vi "Create Channel Configuration.vi"(4 "non-random type (DBL)":T1=enum."DBL", 6 "random types? (F)":bool, 7 "base channel name (channel)":string="channel", 11 "channel count":i32) -> (2 "buffer size":u64, 3 "channel configurations":T2[](array[typedef]) {"buffer offset" format="%d bytes"})   [LabVIEW 2017]
uses:
  Builds/Data Sharing Framework/Current/Data Sharing Framework Core/DSF Core.lvlibp/DSF Configuration API/Public/Controls/DSF Engine Channel Configuration.ctl
  Builds/Data Sharing Framework/Current/Data Sharing Framework Core/DSF Core.lvlibp/DSF Configuration API/Public/Controls/DSF Data Type.ctl
  Builds/Data Sharing Framework/Current/Data Sharing Framework Core/DSF Core.lvlibp/DSF Configuration API/Public/Controls/DSF Settings Info.ctl
  Builds/Data Sharing Framework/Current/Data Sharing Framework Core/DSF Core.lvlibp
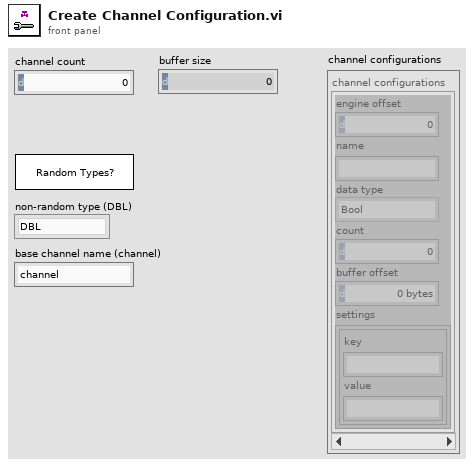
[diagram p1: front panel]
types:
  T1 = typedef "DSF Core.lvlibp/DSF Data Type.ctl" = enum8{"Bool", "SGL", "DBL", "I8", "I16", "I32", "I64", "U8", "U16", "U32", "U64"}
  T2 = typedef "DSF Core.lvlibp/DSF Engine Channel Configuration.ctl" = cluster{"engine offset":u64, "name":string, "data type":T1, "count":u64, "buffer offset":u64, "settings":T3}
  T3 = typedef "DSF Core.lvlibp/DSF Settings Info.ctl" = cluster{"key":string, "value":string}[]
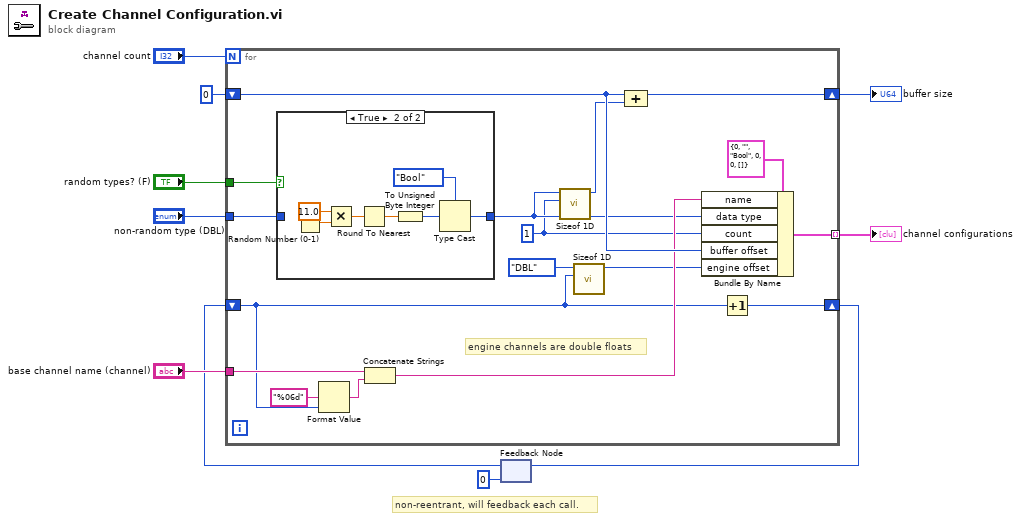
[diagram p0: block diagram]
diagram:
  # "non-reentrant, will feedback each call."
  n1 = feedback #1(u64 0) -> (w3:u64)
  n2 = for {
    N: "channel count" -> [_]
    tunnel: "non-random type (DBL)" -> [w26]
    tunnel: "random types? (F)" -> [w27]
    shift-right: [w25] -> w4
    shift-left: u64 0 ("buffer offset") -> [w24]
    tunnel: "base channel name (channel)" -> [w21]
    tunnel: [w19] -> w5 mode=indexing
    shift-right: [w17] -> w1
    shift-left: w3 -> [w16]
    w12 = u64 1 ("count")
    # "engine channels are double floats"
    n3 = case shown="True" w27 {
      tunnel: [w28 w30] -> w13
      tunnel: w26 -> [w28 _]
      frame False {
      }
      frame True {
        n4 = Random Number (0-1)() -> (number: 0 to 1=w34:dbl)
        n5 = Multiply(x=11.0, y=w34) -> (x*y=w31:dbl)
        n6 = Round To Nearest(number=w31) -> (nearest integer value=w35:dbl)
        n7 = To Unsigned Byte Integer(number=w35) -> (unsigned 8bit integer=w32:u8)
        n8 = Type Cast(type=DSF_Data_Type."Bool" ("data type"), x=w32) -> (*(type *) &x=w30:T1)
      }
    }
    n9 = Format Value(format string="%06d", value (0)=w16) -> (output string=w23:string)  [unwired: 1 in]
    n10 = Concatenate Strings(w21, w23) -> (w20:string)
    n11 = call "Sizeof 1D.vi"("count"=w12, "data type"=w13) -> ("size in bytes"=w11:u64)  [unwired: 9 in]
    n12 = call "Sizeof 1D.vi"("count"=w16, "data type"=DSF_Data_Type."DBL") -> ("size in bytes"=w15:u64)  [unwired: 9 in]
    n13 = Compound Arithmetic op=ADD(w24, w11) -> (w25:u64)
    n14 = Bundle By Name(cluster=T2 {"engine offset"=0, "name"="", "data type"=enum."Bool", "count"=0, "buffer offset"=0, "settings"=[]} ("channel configurations"), "name"=w20, "data type"=w13, "count"=w12, "buffer offset"=w24, "engine offset"=w15) -> (w19:T2)
    n15 = Increment(x=w16) -> (x+1=w17:u64)
  }
  "channel configurations" <- w5
  "buffer size" <- w4
  n16 = feedback-in #1(w1) -> ()
